vi "Instructor.vi"() -> ()   [LabVIEW 2017]
uses:
  <vilib>/Analysis/baseanly.llb/Mean (DBL).vi
  <vilib>/Utility/file.llb/Read Delimited Spreadsheet (DBL).vi
  <vilib>/Analysis/NI_AALBase.lvlib
panel:
  in  "error in (no error)":errorcluster
  in  "Desired Power":bool
  in  "Desired Power_S":sgl format="%#.1f"
  in  "TCHXActive":bool
  in  "PowerActive":bool
  in  "CTAHActive":bool
  in  "PumpActive":bool
  in  "ACTIVATE - TCHX_S":bool
  in  "ACTIVATE - PUMP_S":bool
  in  "ACTIVATE - CTAH_S":bool
  in  "Power Output On_S":bool
  in  "TCHXFreq_S":sgl format="%#.1f"
  in  "TCHXFreq":bool
  in  "Power_S":sgl format="%#.1f"
  in  "Power":bool
  in  "CTAHFreq_S":sgl format="%#.1f"
  in  "CTAHFreq":bool
  in  "PumpFreq_S":sgl format="%#.1f"
  in  "PumpFreq":bool
  out "W":sgl format="%.1f"
  out "S":sgl format="%.1f"
  out "E":sgl format="%.1f"
  out "N":sgl format="%.1f"
  out "SW":sgl format="%.1f"
  out "SE":sgl format="%.1f"
  out "N":sgl format="%.1f"
  out "Server Connection":bool
  in  "B66":bool
  in  "W67":bool
  in  "B60":bool
  in  "W61":bool
  in  "B65":bool
  in  "W64":bool
  in  "B21":bool
  in  "W20":bool
  in  "B23":bool
  in  "W22":bool
  in  "B63":bool
  in  "W62":bool
  in  "A01":bool
  in  "A02":bool
  in  "W24":bool
  in  "B25":bool
  in  "W26":bool
  in  "B27":bool
  in  "B12":bool
  in  "W13":bool
  in  "C11":bool
  in  "C10":bool
  in  "S13":bool
  in  "S11":bool
  in  "S10":bool
  in  "W35":bool
  in  "B34":bool
  in  "B43":bool
  in  "W42":bool
  in  "W40":bool
  in  "B41":bool
  in  "W33":bool
  in  "B32":bool
  in  "W31":bool
  in  "B30":bool
  in  "W10":bool
  in  "B11":bool
  in  "B29":bool
  in  "W28":bool
  in  "Spoof Enabled":bool
  in  "Stop Instructor":bool
  in  "BT-63_S":sgl format="%.1g"
  in  "WT-35_S":sgl format="%.1g"
  in  "BT-34_S":sgl format="%.1g"
  in  "ST-13_S":sgl format="%.1g"
  in  "ST-11_S":sgl format="%.1g"
  in  "ST-10_S":sgl format="%.1g"
  in  "BT-29_S":sgl format="%.1g"
  in  "BT-60_S":sgl format="%.1g"
  in  "AT-02_S":sgl format="%.1g"
  in  "AT-01_S":sgl format="%.1g"
  in  "BT-30_S":sgl format="%.1g"
  in  "BT-66_S":sgl format="%.1g"
  in  "BT-65_S":sgl format="%.1g"
  in  "BT-21_S":sgl format="%.1g"
  in  "BT-23_S":sgl format="%.1g"
  in  "BT-25_S":sgl format="%.1g"
  in  "BT-27_S":sgl format="%.1g"
  in  "BT-32_S":sgl format="%.1g"
  in  "BT-43_S":sgl format="%.1g"
  in  "BT-41_S":sgl format="%.1g"
  in  "WT-67_S":sgl format="%.1g"
  in  "WT-61_S":sgl format="%.1g"
  in  "WT-64_S":sgl format="%.1g"
  in  "WT-62_S":sgl format="%.1g"
  in  "WT-20_S":sgl format="%.1g"
  in  "WT-22_S":sgl format="%.1g"
  in  "WT-33_S":sgl format="%.1g"
  in  "WT-24_S":sgl format="%.1g"
  in  "WT-26_S":sgl format="%.1g"
  in  "WT-28_S":sgl format="%.1g"
  in  "WT-42_S":sgl format="%.1g"
  in  "WT-40_S":sgl format="%.1g"
  in  "WT-31_S":sgl format="%.1g"
  in  "BT-12_S":sgl format="%.1g"
  in  "BT-11_S":sgl format="%.1g"
  in  "WT-10_S":sgl format="%.1g"
  in  "CX-11_S":sgl format="%.1g"
  in  "CX-10_S":sgl format="%.1g"
  out "DRACS Flow\n\n\nFM-60 [kg/s]":sgl format="%.3f"
  out "Primary Flow\n\n\nFM-40 [kg/s]":sgl format="%.3f"
  out "Bypass Flow\n\n\nFM-30 [kg/s]":sgl format="%.3f"
  out "DHX Primary Flow\n\n\nFM-20 [kg/s]":sgl format="%.3f"
  out "AT-02":sgl format="%.1g"
  out "AT-01":sgl format="%.1g"
  out "ST-13":sgl format="%.1f"
  out "ST-11":sgl format="%.1f"
  out "ST-10":sgl format="%.1f"
  out "WT-67":sgl format="%.1f"
  out "BT-66":sgl format="%.1f"
  out "BT-65":sgl format="%.1f"
  out "WT-64":sgl format="%.1f"
  out "BT-63":sgl format="%.1f"
  out "WT-62":sgl format="%.1f"
  out "WT-61":sgl format="%.1f"
  out "BT-60":sgl format="%.1f"
  out "BT-43":sgl format="%.1g"
  out "WT-42":sgl format="%.1g"
  out "BT-41":sgl format="%.1g"
  out "WT-40":sgl format="%.1g"
  out "WT-35":sgl format="%.1g"
  out "BT-34":sgl format="%.1g"
  out "WT-33":sgl format="%.1g"
  out "BT-32":sgl format="%.1g"
  out "WT-31":sgl format="%.1g"
  out "BT-30":sgl format="%.1g"
  out "BT-29":sgl format="%.1f"
  out "WT-28":sgl format="%.1f"
  out "BT-27":sgl format="%.1f"
  out "WT-26":sgl format="%.1f"
  out "BT-25":sgl format="%.1f"
  out "WT-24":sgl format="%.1f"
  out "BT-23":sgl format="%.1f"
  out "WT-22":sgl format="%.1f"
  out "BT-21":sgl format="%.1f"
  out "WT-20":sgl format="%.1f"
  out "CX-11":sgl format="%.1g"
  out "CX-10":sgl format="%.1g"
  out "WT-13":sgl format="%.1g"
  out "BT-12":sgl format="%.1g"
  out "BT-11":sgl format="%.1g"
  out "WT-10":sgl format="%.1g"
  out "Power [W]":sgl(slide) caption="Power Output [W]" scale=0.0..10000.0
  out "Frequency [Hz]":sgl(knob) scale=0.0..45.0
  out "Frequency [Hz] 3":sgl(slide) scale=0.0..60.0
  out "Frequency [Hz]":sgl(slide) scale=0.0..60.0
  in  "WT-13_S":sgl format="%.1g"
  out "Power Output":sgl(graph)
  out "System Safe":bool
  out "System Time [s]":sgl format="%#.1f"
  out "System Loop Time (ms)":u32
  in  "Load Power Profile":bool
  in  "Dyn. Power Profile File":path
  out "CTAH Temperatures":cluster{"CTAH Outlet":dbl, "CTAH Inlet":dbl}(graph)
  out "CTAH Outlet":dbl format="%0.2f"
  out "CTAH Inlet":dbl format="%0.2f"
  out "Core Temperatures":cluster{"Heater Inlet":dbl, "Heater Outlet":dbl}(graph)
  out "Heater Outlet":dbl format="%0.2f"
  out "Heater Inlet":dbl format="%0.2f"
  out "Profile Step":i32
  out "Power Input Signal [W]":dbl
  out "Output Current 2 [A]":dbl
  out "Output Voltage 2 [V]":dbl
  out "Output Current 1 [A]":dbl
  out "Output Voltage 1 [V]":dbl
  out "Loop Period [ms]":i64
  # "System Analytics"
  # "DRACS"
  # "PRIMARY"
  # "HOT DRACS"
  # "DHX TOP"
  # "TCHX"
  # "HOT LEG"
  # "DHX"
  # "COLD DRACS"
  # "ST-14"
  # "BYPASS"
  # "CTAH"
  # "ST-12"
  # "DHX BOTTOM"
  # "HEATER"
  # "COLD LEG"
  # "PUMP"
  # "Action Log"
  # "Action Log Box"
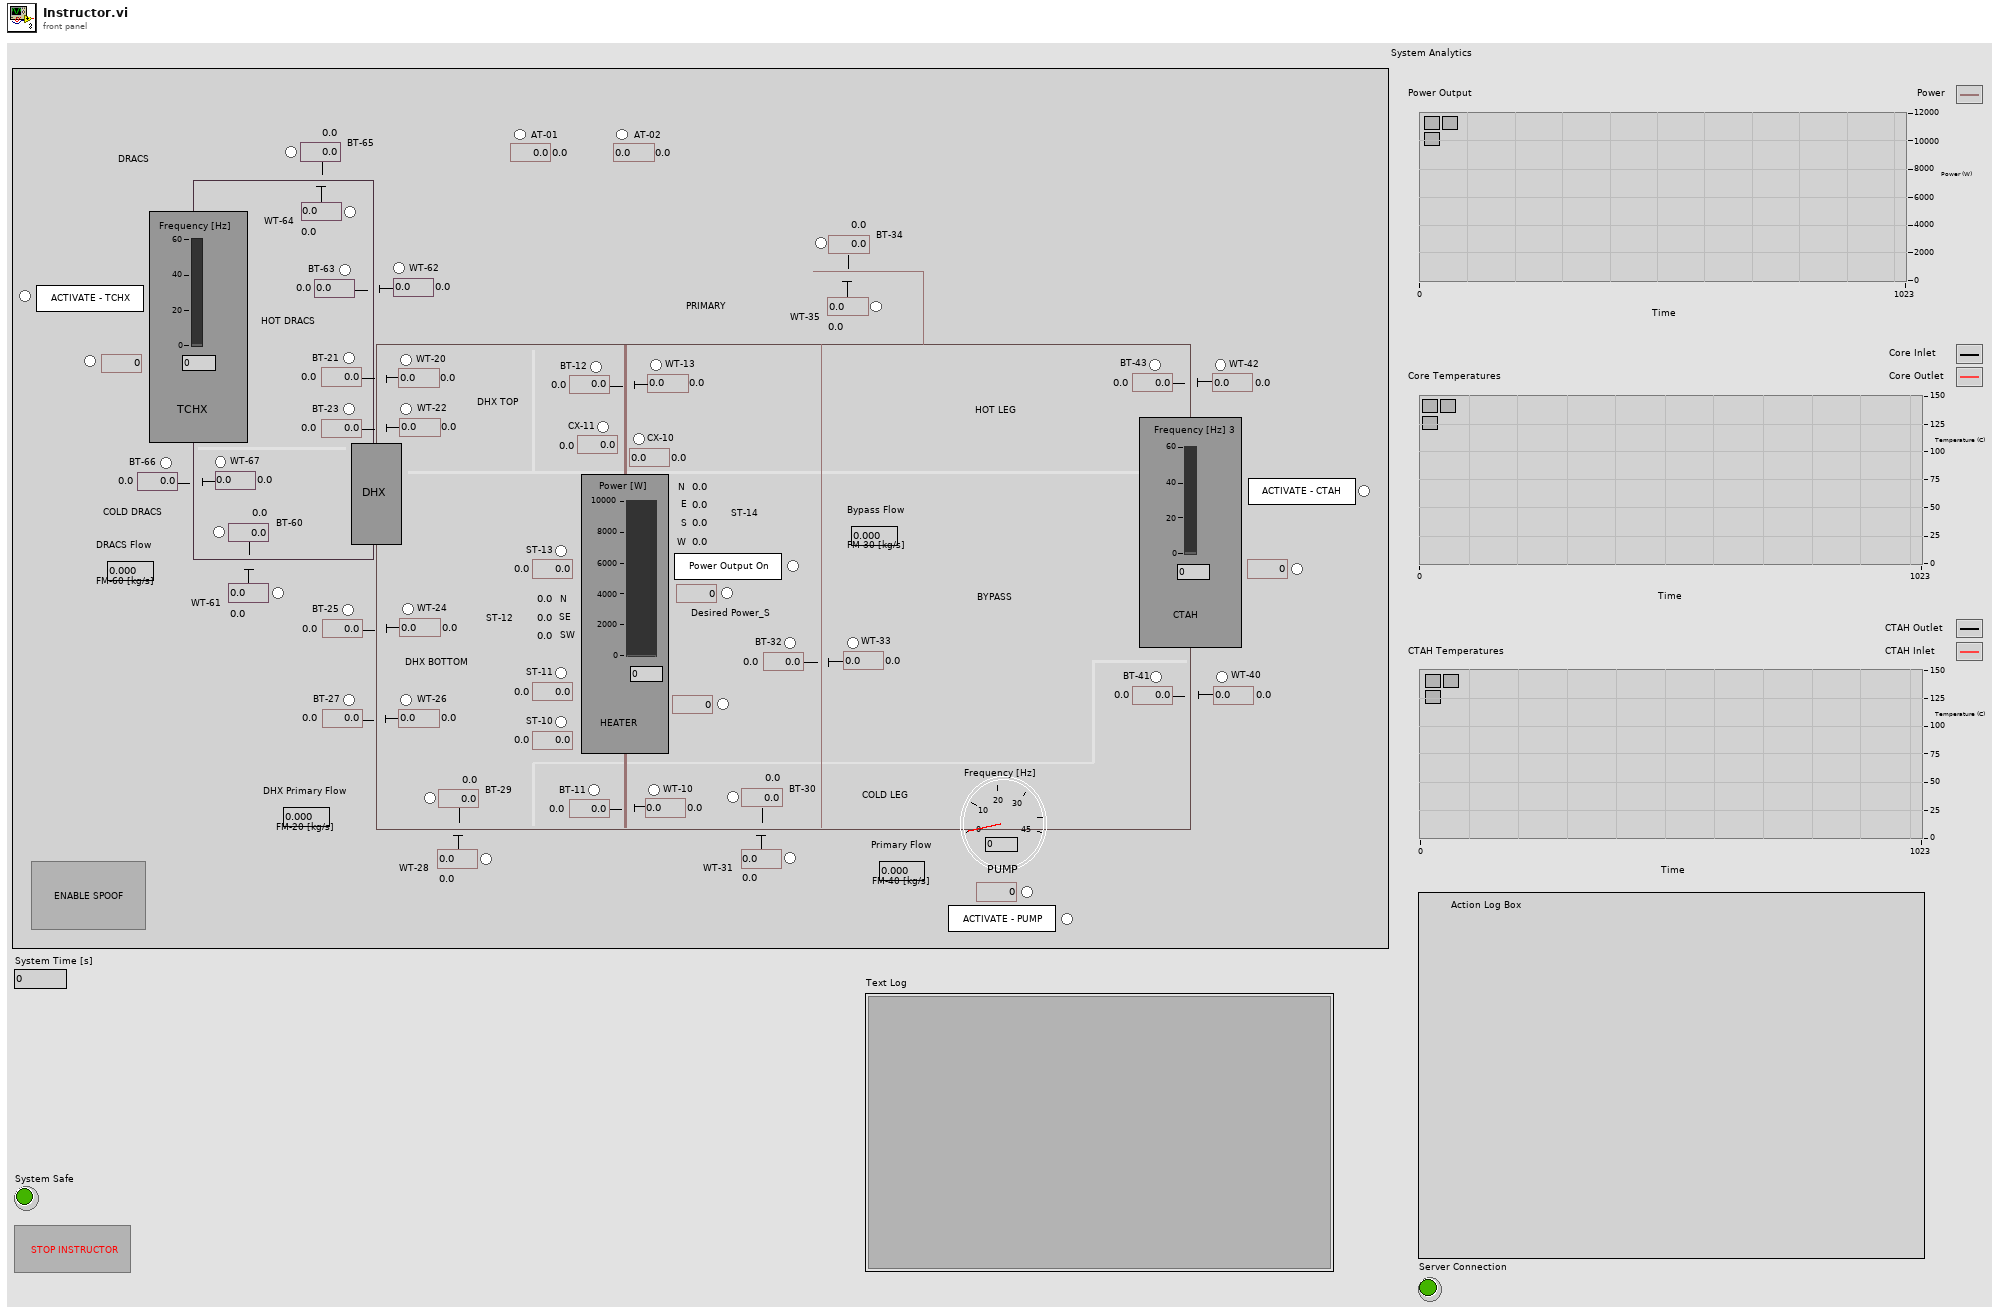
[diagram p1: front panel]
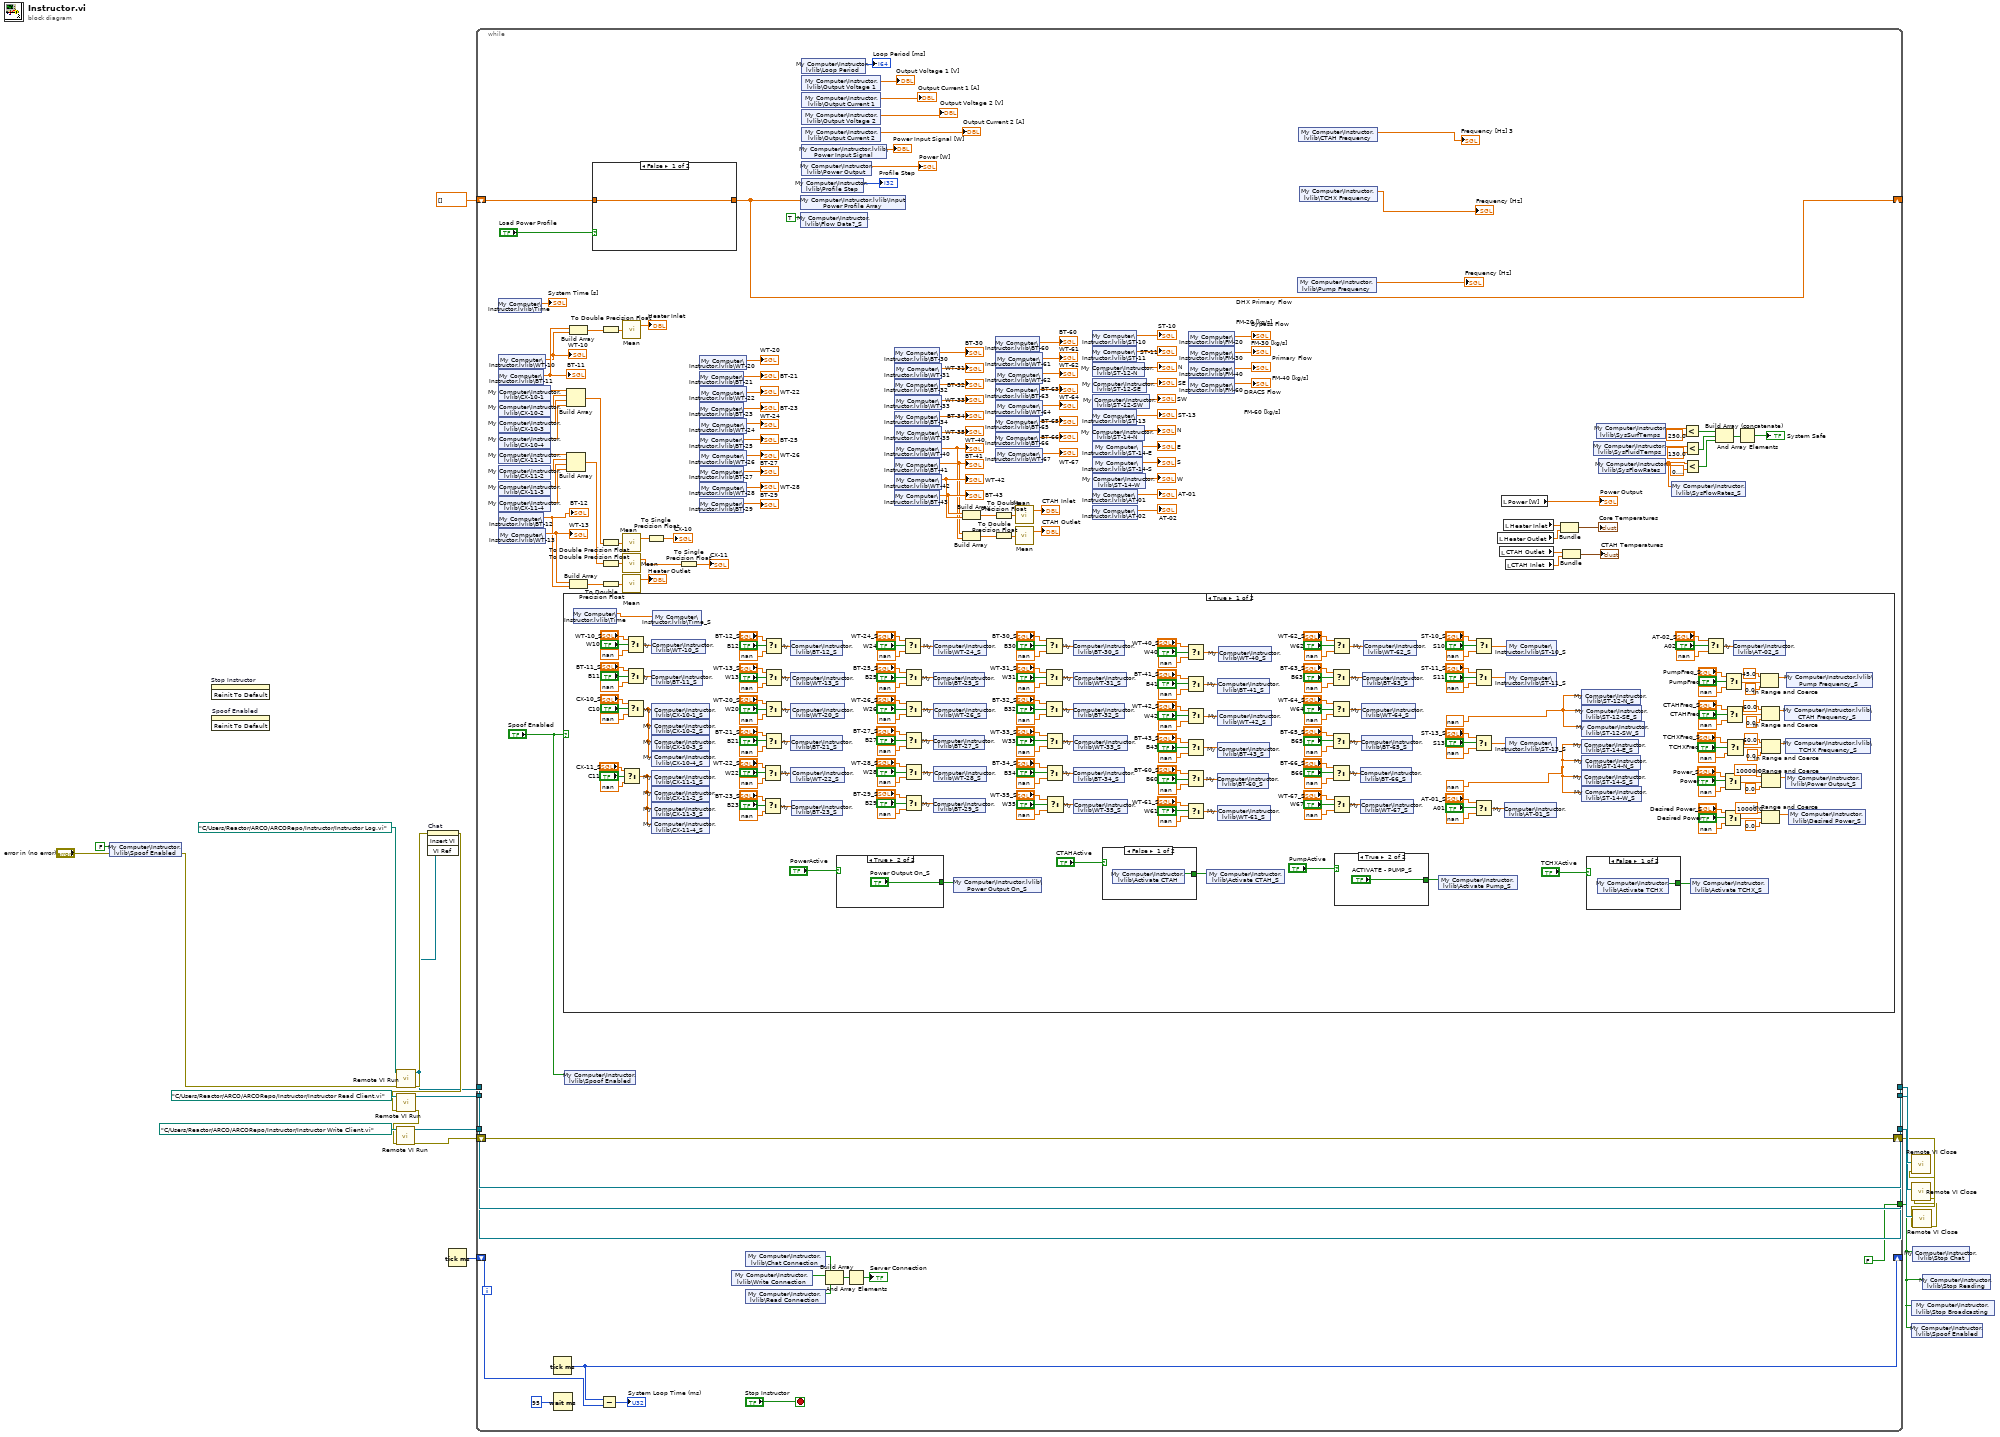
[diagram p0: block diagram]
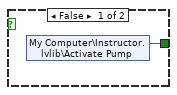
[diagram p2: hidden frame]
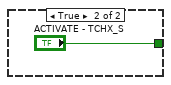
[diagram p3: hidden frame]
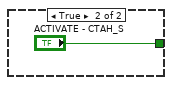
[diagram p4: hidden frame]
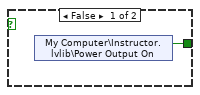
[diagram p5: hidden frame]
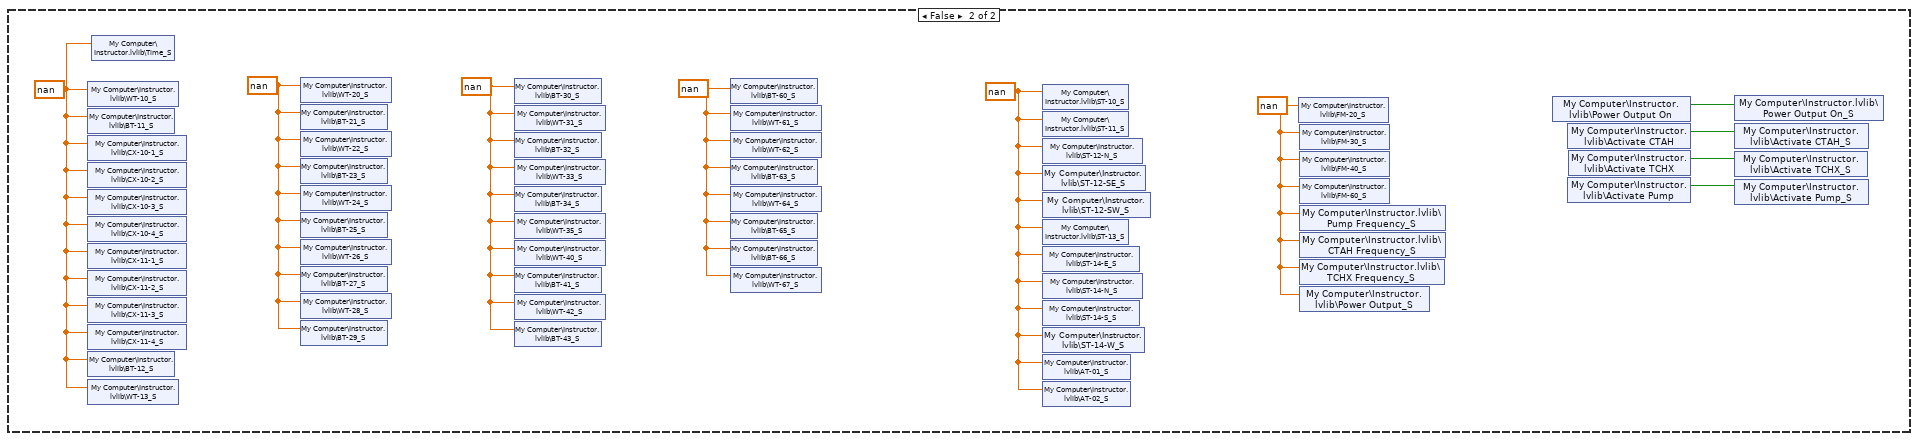
[diagram p6: hidden frame]
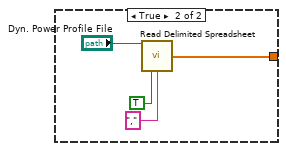
[diagram p7: hidden frame]
diagram:
  n1 = shared-variable "My Computer\\Instructor.lvlib\\Spoof Enabled"(FALSE ("Spoof Enabled"), error in="error in (no error)") -> (error out=w10:errorcluster)
  n2 = invoke on="Stop Instructor" class="Bool (strict)" method="Reinit To Default"() -> ()  [unwired: 3 in, 3 out]
  n3 = invoke on="Spoof Enabled" class="Bool (strict)" method="Reinit To Default"() -> ()  [unwired: 3 in, 3 out]
  n4 = call "Remote VI Run.vi"("error in (no error)"=w10, "VI Path"=path "C:/Users/Reactor/ARCO/ARCORepo/Instructor/Instructor Log.vi" ("vi path")) -> ("error out"=w9:errorcluster, "VI Reference"=w7:refnum<vi>)  [unwired: 8 in]
  n5 = invoke on="Chat" class="SubPnl" method="Insert VI"(error in=w9, "VI Ref"=w7) -> (error out=w8:errorcluster)  [unwired: 2 in, 3 out]
  n6 = call "Remote VI Run.vi"("error in (no error)"=w8, "VI Path"=path "C:/Users/Reactor/ARCO/ARCORepo/Instructor/Instructor Read Client.vi") -> ("error out"=w6:errorcluster, "VI Reference"=w18:refnum<vi>)  [unwired: 8 in]
  n7 = call "Remote VI Run.vi"("error in (no error)"=w6, "VI Path"=path "C:/Users/Reactor/ARCO/ARCORepo/Instructor/Instructor Write Client.vi") -> ("error out"=w5:errorcluster, "VI Reference"=w14:refnum<vi>)  [unwired: 8 in]
  n8 = Tick Count (ms)() -> (millisecond timer value=w21:u32)
  n9 = while {
    shift-right: [w73] -> _
    shift-left: dbl[] [] ("Input Power Profile Array") -> [w74]
    shift-right: [w71] -> _
    shift-left: w21 -> [w72]
    tunnel: w7 -> [w45]
    tunnel: w18 -> [w44]
    tunnel: [w45] -> w17
    tunnel: [w44] -> w16
    tunnel: w14 -> [w43]
    tunnel: [w43] -> w13
    tunnel: [FALSE] -> w12
    shift-right: [w24] -> w4
    shift-left: w5 -> [w24]
    stop <- "Stop Instructor" stop-if-true
    n10 = shared-variable "My Computer\\Instructor.lvlib\\Time"() -> (→"System Time [s]":sgl)  [unwired: 1 in, 1 out]
    n11 = shared-variable "My Computer\\Instructor.lvlib\\WT-10"() -> (w52:sgl)  [unwired: 1 in, 1 out]
    "WT-10" <- w52
    n12 = shared-variable "My Computer\\Instructor.lvlib\\BT-11"() -> (w56:sgl)  [unwired: 1 in, 1 out]
    "BT-11" <- w56
    n13 = shared-variable "My Computer\\Instructor.lvlib\\CX-10-1"() -> (w139:sgl)  [unwired: 1 in, 1 out]
    n14 = shared-variable "My Computer\\Instructor.lvlib\\CX-10-2"() -> (w138:sgl)  [unwired: 1 in, 1 out]
    n15 = shared-variable "My Computer\\Instructor.lvlib\\CX-10-3"() -> (w137:sgl)  [unwired: 1 in, 1 out]
    n16 = shared-variable "My Computer\\Instructor.lvlib\\CX-10-4"() -> (w136:sgl)  [unwired: 1 in, 1 out]
    n17 = shared-variable "My Computer\\Instructor.lvlib\\CX-11-1"() -> (w132:sgl)  [unwired: 1 in, 1 out]
    n18 = shared-variable "My Computer\\Instructor.lvlib\\CX-11-2"() -> (w131:sgl)  [unwired: 1 in, 1 out]
    n19 = shared-variable "My Computer\\Instructor.lvlib\\CX-11-3"() -> (w130:sgl)  [unwired: 1 in, 1 out]
    n20 = shared-variable "My Computer\\Instructor.lvlib\\CX-11-4"() -> (w129:sgl)  [unwired: 1 in, 1 out]
    n21 = shared-variable "My Computer\\Instructor.lvlib\\BT-12"() -> (w55:sgl)  [unwired: 1 in, 1 out]
    "BT-12" <- w55
    n22 = shared-variable "My Computer\\Instructor.lvlib\\WT-13"() -> (w96:sgl)  [unwired: 1 in, 1 out]
    "WT-13" <- w96
    n23 = Tick Count (ms)() -> (millisecond timer value=w71:u32)
    n24 = Wait (ms)(milliseconds to wait=u32 95) -> ()  [unwired: 1 out]
    n25 = case shown="True" "Spoof Enabled" {
      frame True {
        w192 = sgl nan
        w193 = sgl nan
        n26 = shared-variable "My Computer\\Instructor.lvlib\\Time"() -> (w194:sgl)  [unwired: 1 in, 1 out]
        n27 = Select(t="CX-11_S", s="C11", f=sgl nan) -> (s? t:f=w335:sgl)
        n28 = Select(t="WT-10_S", s="W10", f=sgl nan) -> (s? t:f=w347:sgl)
        n29 = Select(t="BT-11_S", s="B11", f=sgl nan) -> (s? t:f=w343:sgl)
        n30 = Select(t="CX-10_S", s="C10", f=sgl nan) -> (s? t:f=w339:sgl)
        n31 = shared-variable "My Computer\\Instructor.lvlib\\WT-10_S"(w347) -> ()  [unwired: 1 in, 1 out]
        n32 = shared-variable "My Computer\\Instructor.lvlib\\BT-11_S"(w343) -> ()  [unwired: 1 in, 1 out]
        n33 = shared-variable "My Computer\\Instructor.lvlib\\CX-10-1_S"(w339) -> ()  [unwired: 1 in, 1 out]
        n34 = shared-variable "My Computer\\Instructor.lvlib\\CX-10-2_S"(w339) -> ()  [unwired: 1 in, 1 out]
        n35 = shared-variable "My Computer\\Instructor.lvlib\\CX-10-3_S"(w339) -> ()  [unwired: 1 in, 1 out]
        n36 = shared-variable "My Computer\\Instructor.lvlib\\CX-10-4_S"(w339) -> ()  [unwired: 1 in, 1 out]
        n37 = shared-variable "My Computer\\Instructor.lvlib\\CX-11-1_S"(w335) -> ()  [unwired: 1 in, 1 out]
        n38 = shared-variable "My Computer\\Instructor.lvlib\\CX-11-2_S"(w335) -> ()  [unwired: 1 in, 1 out]
        n39 = shared-variable "My Computer\\Instructor.lvlib\\CX-11-3_S"(w335) -> ()  [unwired: 1 in, 1 out]
        n40 = shared-variable "My Computer\\Instructor.lvlib\\CX-11-4_S"(w335) -> ()  [unwired: 1 in, 1 out]
        n41 = shared-variable "My Computer\\Instructor.lvlib\\Time_S"(w194) -> ()  [unwired: 1 in, 1 out]
        n42 = Select(t="WT-22_S", s="W22", f=sgl nan) -> (s? t:f=w315:sgl)
        n43 = Select(t="BT-23_S", s="B23", f=sgl nan) -> (s? t:f=w311:sgl)
        n44 = Select(t="BT-12_S", s="B12", f=sgl nan) -> (s? t:f=w331:sgl)
        n45 = Select(t="WT-13_S", s="W13", f=sgl nan) -> (s? t:f=w327:sgl)
        n46 = Select(t="WT-20_S", s="W20", f=sgl nan) -> (s? t:f=w323:sgl)
        n47 = Select(t="BT-21_S", s="B21", f=sgl nan) -> (s? t:f=w319:sgl)
        n48 = shared-variable "My Computer\\Instructor.lvlib\\BT-12_S"(w331) -> ()  [unwired: 1 in, 1 out]
        n49 = shared-variable "My Computer\\Instructor.lvlib\\WT-13_S"(w327) -> ()  [unwired: 1 in, 1 out]
        n50 = shared-variable "My Computer\\Instructor.lvlib\\WT-20_S"(w323) -> ()  [unwired: 1 in, 1 out]
        n51 = shared-variable "My Computer\\Instructor.lvlib\\BT-21_S"(w319) -> ()  [unwired: 1 in, 1 out]
        n52 = shared-variable "My Computer\\Instructor.lvlib\\WT-22_S"(w315) -> ()  [unwired: 1 in, 1 out]
        n53 = shared-variable "My Computer\\Instructor.lvlib\\BT-23_S"(w311) -> ()  [unwired: 1 in, 1 out]
        n54 = case shown="True" "PowerActive" {
          tunnel: [w357 "Power Output On_S"] -> w155
          frame False {
            n55 = shared-variable "My Computer\\Instructor.lvlib\\Power Output On"() -> (w357:bool)  [unwired: 1 in, 1 out]
          }
          frame True {
          }
        }
        n56 = Select(t="WT-24_S", s="W24", f=sgl nan) -> (s? t:f=w307:sgl)
        n57 = Select(t="BT-25_S", s="B25", f=sgl nan) -> (s? t:f=w303:sgl)
        n58 = Select(t="WT-26_S", s="W26", f=sgl nan) -> (s? t:f=w299:sgl)
        n59 = Select(t="BT-27_S", s="B27", f=sgl nan) -> (s? t:f=w295:sgl)
        n60 = Select(t="WT-28_S", s="W28", f=sgl nan) -> (s? t:f=w291:sgl)
        n61 = Select(t="BT-29_S", s="B29", f=sgl nan) -> (s? t:f=w287:sgl)
        n62 = shared-variable "My Computer\\Instructor.lvlib\\WT-24_S"(w307) -> ()  [unwired: 1 in, 1 out]
        n63 = shared-variable "My Computer\\Instructor.lvlib\\BT-25_S"(w303) -> ()  [unwired: 1 in, 1 out]
        n64 = shared-variable "My Computer\\Instructor.lvlib\\WT-26_S"(w299) -> ()  [unwired: 1 in, 1 out]
        n65 = shared-variable "My Computer\\Instructor.lvlib\\BT-27_S"(w295) -> ()  [unwired: 1 in, 1 out]
        n66 = shared-variable "My Computer\\Instructor.lvlib\\WT-28_S"(w291) -> ()  [unwired: 1 in, 1 out]
        n67 = shared-variable "My Computer\\Instructor.lvlib\\BT-29_S"(w287) -> ()  [unwired: 1 in, 1 out]
        n68 = shared-variable "My Computer\\Instructor.lvlib\\Power Output On_S"(w155) -> ()  [unwired: 1 in, 1 out]
        n69 = Select(t="BT-30_S", s="B30", f=sgl nan) -> (s? t:f=w283:sgl)
        n70 = Select(t="WT-31_S", s="W31", f=sgl nan) -> (s? t:f=w279:sgl)
        n71 = Select(t="BT-32_S", s="B32", f=sgl nan) -> (s? t:f=w275:sgl)
        n72 = Select(t="WT-33_S", s="W33", f=sgl nan) -> (s? t:f=w271:sgl)
        n73 = Select(t="BT-34_S", s="B34", f=sgl nan) -> (s? t:f=w267:sgl)
        n74 = Select(t="WT-35_S", s="W35", f=sgl nan) -> (s? t:f=w263:sgl)
        n75 = shared-variable "My Computer\\Instructor.lvlib\\WT-31_S"(w279) -> ()  [unwired: 1 in, 1 out]
        n76 = shared-variable "My Computer\\Instructor.lvlib\\BT-32_S"(w275) -> ()  [unwired: 1 in, 1 out]
        n77 = shared-variable "My Computer\\Instructor.lvlib\\BT-30_S"(w283) -> ()  [unwired: 1 in, 1 out]
        n78 = shared-variable "My Computer\\Instructor.lvlib\\WT-33_S"(w271) -> ()  [unwired: 1 in, 1 out]
        n79 = shared-variable "My Computer\\Instructor.lvlib\\BT-34_S"(w267) -> ()  [unwired: 1 in, 1 out]
        n80 = shared-variable "My Computer\\Instructor.lvlib\\WT-35_S"(w263) -> ()  [unwired: 1 in, 1 out]
        n81 = case shown="False" "CTAHActive" {
          tunnel: [w355 "ACTIVATE - CTAH_S"] -> w153
          frame False {
            n82 = shared-variable "My Computer\\Instructor.lvlib\\Activate CTAH"() -> (w355:bool)  [unwired: 1 in, 1 out]
          }
          frame True {
          }
        }
        n83 = Select(t="WT-40_S", s="W40", f=sgl nan) -> (s? t:f=w259:sgl)
        n84 = Select(t="BT-41_S", s="B41", f=sgl nan) -> (s? t:f=w255:sgl)
        n85 = Select(t="WT-42_S", s="W42", f=sgl nan) -> (s? t:f=w251:sgl)
        n86 = Select(t="BT-43_S", s="B43", f=sgl nan) -> (s? t:f=w247:sgl)
        n87 = Select(t="BT-60_S", s="B60", f=sgl nan) -> (s? t:f=w243:sgl)
        n88 = Select(t="WT-61_S", s="W61", f=sgl nan) -> (s? t:f=w239:sgl)
        n89 = shared-variable "My Computer\\Instructor.lvlib\\Activate CTAH_S"(w153) -> ()  [unwired: 1 in, 1 out]
        n90 = shared-variable "My Computer\\Instructor.lvlib\\BT-60_S"(w243) -> ()  [unwired: 1 in, 1 out]
        n91 = shared-variable "My Computer\\Instructor.lvlib\\WT-61_S"(w239) -> ()  [unwired: 1 in, 1 out]
        n92 = shared-variable "My Computer\\Instructor.lvlib\\BT-41_S"(w255) -> ()  [unwired: 1 in, 1 out]
        n93 = shared-variable "My Computer\\Instructor.lvlib\\WT-42_S"(w251) -> ()  [unwired: 1 in, 1 out]
        n94 = shared-variable "My Computer\\Instructor.lvlib\\BT-43_S"(w247) -> ()  [unwired: 1 in, 1 out]
        n95 = shared-variable "My Computer\\Instructor.lvlib\\WT-40_S"(w259) -> ()  [unwired: 1 in, 1 out]
        n96 = Select(t="BT-63_S", s="B63", f=sgl nan) -> (s? t:f=w231:sgl)
        n97 = Select(t="WT-64_S", s="W64", f=sgl nan) -> (s? t:f=w227:sgl)
        n98 = Select(t="BT-65_S", s="B65", f=sgl nan) -> (s? t:f=w223:sgl)
        n99 = Select(t="BT-66_S", s="B66", f=sgl nan) -> (s? t:f=w219:sgl)
        n100 = Select(t="WT-62_S", s="W62", f=sgl nan) -> (s? t:f=w235:sgl)
        n101 = Select(t="WT-67_S", s="W67", f=sgl nan) -> (s? t:f=w215:sgl)
        n102 = case shown="True" "PumpActive" {
          tunnel: [w351 "ACTIVATE - PUMP_S"] -> w149
          frame False {
            n103 = shared-variable "My Computer\\Instructor.lvlib\\Activate Pump"() -> (w351:bool)  [unwired: 1 in, 1 out]
          }
          frame True {
          }
        }
        n104 = shared-variable "My Computer\\Instructor.lvlib\\WT-67_S"(w215) -> ()  [unwired: 1 in, 1 out]
        n105 = shared-variable "My Computer\\Instructor.lvlib\\BT-66_S"(w219) -> ()  [unwired: 1 in, 1 out]
        n106 = shared-variable "My Computer\\Instructor.lvlib\\BT-65_S"(w223) -> ()  [unwired: 1 in, 1 out]
        n107 = shared-variable "My Computer\\Instructor.lvlib\\WT-64_S"(w227) -> ()  [unwired: 1 in, 1 out]
        n108 = shared-variable "My Computer\\Instructor.lvlib\\BT-63_S"(w231) -> ()  [unwired: 1 in, 1 out]
        n109 = shared-variable "My Computer\\Instructor.lvlib\\WT-62_S"(w235) -> ()  [unwired: 1 in, 1 out]
        n110 = shared-variable "My Computer\\Instructor.lvlib\\Activate Pump_S"(w149) -> ()  [unwired: 1 in, 1 out]
        n111 = Select(t="ST-11_S", s="S11", f=sgl nan) -> (s? t:f=w207:sgl)
        n112 = Select(t="ST-13_S", s="S13", f=sgl nan) -> (s? t:f=w203:sgl)
        n113 = Select(t="AT-01_S", s="A01", f=sgl nan) -> (s? t:f=w199:sgl)
        n114 = Select(t="ST-10_S", s="S10", f=sgl nan) -> (s? t:f=w211:sgl)
        n115 = shared-variable "My Computer\\Instructor.lvlib\\AT-01_S"(w199) -> ()  [unwired: 1 in, 1 out]
        n116 = shared-variable "My Computer\\Instructor.lvlib\\ST-11_S"(w207) -> ()  [unwired: 1 in, 1 out]
        n117 = shared-variable "My Computer\\Instructor.lvlib\\ST-13_S"(w203) -> ()  [unwired: 1 in, 1 out]
        n118 = shared-variable "My Computer\\Instructor.lvlib\\ST-10_S"(w211) -> ()  [unwired: 1 in, 1 out]
        n119 = shared-variable "My Computer\\Instructor.lvlib\\ST-12-N_S"(w193) -> ()  [unwired: 1 in, 1 out]
        n120 = shared-variable "My Computer\\Instructor.lvlib\\ST-12-SE_S"(w193) -> ()  [unwired: 1 in, 1 out]
        n121 = shared-variable "My Computer\\Instructor.lvlib\\ST-12-SW_S"(w193) -> ()  [unwired: 1 in, 1 out]
        n122 = shared-variable "My Computer\\Instructor.lvlib\\ST-14-E_S"(w192) -> ()  [unwired: 1 in, 1 out]
        n123 = shared-variable "My Computer\\Instructor.lvlib\\ST-14-N_S"(w192) -> ()  [unwired: 1 in, 1 out]
        n124 = shared-variable "My Computer\\Instructor.lvlib\\ST-14-S_S"(w192) -> ()  [unwired: 1 in, 1 out]
        n125 = shared-variable "My Computer\\Instructor.lvlib\\ST-14-W_S"(w192) -> ()  [unwired: 1 in, 1 out]
        n126 = case shown="False" "TCHXActive" {
          tunnel: [w353 "ACTIVATE - TCHX_S"] -> w151
          frame False {
            n127 = shared-variable "My Computer\\Instructor.lvlib\\Activate TCHX"() -> (w353:bool)  [unwired: 1 in, 1 out]
          }
          frame True {
          }
        }
        n128 = shared-variable "My Computer\\Instructor.lvlib\\Activate TCHX_S"(w151) -> ()  [unwired: 1 in, 1 out]
        n129 = Select(t="AT-02_S", s="A02", f=sgl nan) -> (s? t:f=w195:sgl)
        n130 = Select(t="Power_S", s="Power", f=sgl nan) -> (s? t:f=w164:sgl)
        n131 = Select(t="Desired Power_S", s="Desired Power", f=sgl nan) -> (s? t:f=w161:sgl)
        n132 = Select(t="PumpFreq_S", s="PumpFreq", f=sgl nan) -> (s? t:f=w186:sgl)
        n133 = Select(t="CTAHFreq_S", s="CTAHFreq", f=sgl nan) -> (s? t:f=w182:sgl)
        n134 = Select(t="TCHXFreq_S", s="TCHXFreq", f=sgl nan) -> (s? t:f=w175:sgl)
        n135 = shared-variable "My Computer\\Instructor.lvlib\\AT-02_S"(w195) -> ()  [unwired: 1 in, 1 out]
        n136 = In Range and Coerce(upper limit=sgl 45.0, x=w186, lower limit=sgl 0.0) -> (coerced(x)=w185:sgl)  [unwired: 1 out]
        n137 = In Range and Coerce(upper limit=sgl 60.0, x=w182, lower limit=sgl 0.0) -> (coerced(x)=w178:sgl)  [unwired: 1 out]
        n138 = In Range and Coerce(upper limit=sgl 10000.0, x=w161, lower limit=sgl 0.0) -> (coerced(x)=w160:sgl)  [unwired: 1 out]
        n139 = In Range and Coerce(upper limit=sgl 60.0, x=w175, lower limit=sgl 0.0) -> (coerced(x)=w171:sgl)  [unwired: 1 out]
        n140 = In Range and Coerce(upper limit=sgl 10000.0, x=w164, lower limit=sgl 0.0) -> (coerced(x)=w159:sgl)  [unwired: 1 out]
        n141 = shared-variable "My Computer\\Instructor.lvlib\\CTAH Frequency_S"(w178) -> ()  [unwired: 1 in, 1 out]
        n142 = shared-variable "My Computer\\Instructor.lvlib\\TCHX Frequency_S"(w171) -> ()  [unwired: 1 in, 1 out]
        n143 = shared-variable "My Computer\\Instructor.lvlib\\Power Output_S"(w159) -> ()  [unwired: 1 in, 1 out]
        n144 = shared-variable "My Computer\\Instructor.lvlib\\Pump Frequency_S"(w185) -> ()  [unwired: 1 in, 1 out]
        n145 = shared-variable "My Computer\\Instructor.lvlib\\Desired Power_S"(w160) -> ()  [unwired: 1 in, 1 out]
      }
      frame False {
        w363 = sgl nan
        w365 = sgl nan
        w366 = sgl nan
        w367 = sgl nan
        w368 = sgl nan
        w364 = sgl nan
        n146 = shared-variable "My Computer\\Instructor.lvlib\\WT-10_S"(w364) -> ()  [unwired: 1 in, 1 out]
        n147 = shared-variable "My Computer\\Instructor.lvlib\\BT-11_S"(w364) -> ()  [unwired: 1 in, 1 out]
        n148 = shared-variable "My Computer\\Instructor.lvlib\\CX-10-1_S"(w364) -> ()  [unwired: 1 in, 1 out]
        n149 = shared-variable "My Computer\\Instructor.lvlib\\CX-10-2_S"(w364) -> ()  [unwired: 1 in, 1 out]
        n150 = shared-variable "My Computer\\Instructor.lvlib\\CX-10-3_S"(w364) -> ()  [unwired: 1 in, 1 out]
        n151 = shared-variable "My Computer\\Instructor.lvlib\\CX-10-4_S"(w364) -> ()  [unwired: 1 in, 1 out]
        n152 = shared-variable "My Computer\\Instructor.lvlib\\CX-11-1_S"(w364) -> ()  [unwired: 1 in, 1 out]
        n153 = shared-variable "My Computer\\Instructor.lvlib\\CX-11-2_S"(w364) -> ()  [unwired: 1 in, 1 out]
        n154 = shared-variable "My Computer\\Instructor.lvlib\\CX-11-3_S"(w364) -> ()  [unwired: 1 in, 1 out]
        n155 = shared-variable "My Computer\\Instructor.lvlib\\CX-11-4_S"(w364) -> ()  [unwired: 1 in, 1 out]
        n156 = shared-variable "My Computer\\Instructor.lvlib\\BT-12_S"(w364) -> ()  [unwired: 1 in, 1 out]
        n157 = shared-variable "My Computer\\Instructor.lvlib\\WT-13_S"(w364) -> ()  [unwired: 1 in, 1 out]
        n158 = shared-variable "My Computer\\Instructor.lvlib\\Time_S"(w364) -> ()  [unwired: 1 in, 1 out]
        n159 = shared-variable "My Computer\\Instructor.lvlib\\WT-20_S"(w368) -> ()  [unwired: 1 in, 1 out]
        n160 = shared-variable "My Computer\\Instructor.lvlib\\BT-21_S"(w368) -> ()  [unwired: 1 in, 1 out]
        n161 = shared-variable "My Computer\\Instructor.lvlib\\WT-22_S"(w368) -> ()  [unwired: 1 in, 1 out]
        n162 = shared-variable "My Computer\\Instructor.lvlib\\BT-23_S"(w368) -> ()  [unwired: 1 in, 1 out]
        n163 = shared-variable "My Computer\\Instructor.lvlib\\WT-24_S"(w368) -> ()  [unwired: 1 in, 1 out]
        n164 = shared-variable "My Computer\\Instructor.lvlib\\BT-25_S"(w368) -> ()  [unwired: 1 in, 1 out]
        n165 = shared-variable "My Computer\\Instructor.lvlib\\WT-26_S"(w368) -> ()  [unwired: 1 in, 1 out]
        n166 = shared-variable "My Computer\\Instructor.lvlib\\BT-27_S"(w368) -> ()  [unwired: 1 in, 1 out]
        n167 = shared-variable "My Computer\\Instructor.lvlib\\WT-28_S"(w368) -> ()  [unwired: 1 in, 1 out]
        n168 = shared-variable "My Computer\\Instructor.lvlib\\BT-29_S"(w368) -> ()  [unwired: 1 in, 1 out]
        n169 = shared-variable "My Computer\\Instructor.lvlib\\BT-30_S"(w367) -> ()  [unwired: 1 in, 1 out]
        n170 = shared-variable "My Computer\\Instructor.lvlib\\WT-31_S"(w367) -> ()  [unwired: 1 in, 1 out]
        n171 = shared-variable "My Computer\\Instructor.lvlib\\BT-32_S"(w367) -> ()  [unwired: 1 in, 1 out]
        n172 = shared-variable "My Computer\\Instructor.lvlib\\WT-33_S"(w367) -> ()  [unwired: 1 in, 1 out]
        n173 = shared-variable "My Computer\\Instructor.lvlib\\BT-34_S"(w367) -> ()  [unwired: 1 in, 1 out]
        n174 = shared-variable "My Computer\\Instructor.lvlib\\WT-35_S"(w367) -> ()  [unwired: 1 in, 1 out]
        n175 = shared-variable "My Computer\\Instructor.lvlib\\WT-40_S"(w367) -> ()  [unwired: 1 in, 1 out]
        n176 = shared-variable "My Computer\\Instructor.lvlib\\BT-41_S"(w367) -> ()  [unwired: 1 in, 1 out]
        n177 = shared-variable "My Computer\\Instructor.lvlib\\WT-42_S"(w367) -> ()  [unwired: 1 in, 1 out]
        n178 = shared-variable "My Computer\\Instructor.lvlib\\BT-43_S"(w367) -> ()  [unwired: 1 in, 1 out]
        n179 = shared-variable "My Computer\\Instructor.lvlib\\BT-60_S"(w366) -> ()  [unwired: 1 in, 1 out]
        n180 = shared-variable "My Computer\\Instructor.lvlib\\WT-61_S"(w366) -> ()  [unwired: 1 in, 1 out]
        n181 = shared-variable "My Computer\\Instructor.lvlib\\WT-62_S"(w366) -> ()  [unwired: 1 in, 1 out]
        n182 = shared-variable "My Computer\\Instructor.lvlib\\BT-63_S"(w366) -> ()  [unwired: 1 in, 1 out]
        n183 = shared-variable "My Computer\\Instructor.lvlib\\WT-64_S"(w366) -> ()  [unwired: 1 in, 1 out]
        n184 = shared-variable "My Computer\\Instructor.lvlib\\BT-65_S"(w366) -> ()  [unwired: 1 in, 1 out]
        n185 = shared-variable "My Computer\\Instructor.lvlib\\BT-66_S"(w366) -> ()  [unwired: 1 in, 1 out]
        n186 = shared-variable "My Computer\\Instructor.lvlib\\WT-67_S"(w366) -> ()  [unwired: 1 in, 1 out]
        n187 = shared-variable "My Computer\\Instructor.lvlib\\ST-10_S"(w365) -> ()  [unwired: 1 in, 1 out]
        n188 = shared-variable "My Computer\\Instructor.lvlib\\ST-11_S"(w365) -> ()  [unwired: 1 in, 1 out]
        n189 = shared-variable "My Computer\\Instructor.lvlib\\ST-12-N_S"(w365) -> ()  [unwired: 1 in, 1 out]
        n190 = shared-variable "My Computer\\Instructor.lvlib\\ST-12-SE_S"(w365) -> ()  [unwired: 1 in, 1 out]
        n191 = shared-variable "My Computer\\Instructor.lvlib\\ST-12-SW_S"(w365) -> ()  [unwired: 1 in, 1 out]
        n192 = shared-variable "My Computer\\Instructor.lvlib\\ST-13_S"(w365) -> ()  [unwired: 1 in, 1 out]
        n193 = shared-variable "My Computer\\Instructor.lvlib\\ST-14-E_S"(w365) -> ()  [unwired: 1 in, 1 out]
        n194 = shared-variable "My Computer\\Instructor.lvlib\\ST-14-N_S"(w365) -> ()  [unwired: 1 in, 1 out]
        n195 = shared-variable "My Computer\\Instructor.lvlib\\ST-14-S_S"(w365) -> ()  [unwired: 1 in, 1 out]
        n196 = shared-variable "My Computer\\Instructor.lvlib\\ST-14-W_S"(w365) -> ()  [unwired: 1 in, 1 out]
        n197 = shared-variable "My Computer\\Instructor.lvlib\\AT-01_S"(w365) -> ()  [unwired: 1 in, 1 out]
        n198 = shared-variable "My Computer\\Instructor.lvlib\\AT-02_S"(w365) -> ()  [unwired: 1 in, 1 out]
        n199 = shared-variable "My Computer\\Instructor.lvlib\\FM-20_S"(w363) -> ()  [unwired: 1 in, 1 out]
        n200 = shared-variable "My Computer\\Instructor.lvlib\\FM-30_S"(w363) -> ()  [unwired: 1 in, 1 out]
        n201 = shared-variable "My Computer\\Instructor.lvlib\\FM-40_S"(w363) -> ()  [unwired: 1 in, 1 out]
        n202 = shared-variable "My Computer\\Instructor.lvlib\\FM-60_S"(w363) -> ()  [unwired: 1 in, 1 out]
        n203 = shared-variable "My Computer\\Instructor.lvlib\\Pump Frequency_S"(w363) -> ()  [unwired: 1 in, 1 out]
        n204 = shared-variable "My Computer\\Instructor.lvlib\\CTAH Frequency_S"(w363) -> ()  [unwired: 1 in, 1 out]
        n205 = shared-variable "My Computer\\Instructor.lvlib\\TCHX Frequency_S"(w363) -> ()  [unwired: 1 in, 1 out]
        n206 = shared-variable "My Computer\\Instructor.lvlib\\Power Output_S"(w363) -> ()  [unwired: 1 in, 1 out]
        n207 = shared-variable "My Computer\\Instructor.lvlib\\Power Output On"() -> (w362:bool)  [unwired: 1 in, 1 out]
        n208 = shared-variable "My Computer\\Instructor.lvlib\\Activate CTAH"() -> (w361:bool)  [unwired: 1 in, 1 out]
        n209 = shared-variable "My Computer\\Instructor.lvlib\\Activate Pump"() -> (w359:bool)  [unwired: 1 in, 1 out]
        n210 = shared-variable "My Computer\\Instructor.lvlib\\Activate TCHX"() -> (w360:bool)  [unwired: 1 in, 1 out]
        n211 = shared-variable "My Computer\\Instructor.lvlib\\Power Output On_S"(w362) -> ()  [unwired: 1 in, 1 out]
        n212 = shared-variable "My Computer\\Instructor.lvlib\\Activate CTAH_S"(w361) -> ()  [unwired: 1 in, 1 out]
        n213 = shared-variable "My Computer\\Instructor.lvlib\\Activate TCHX_S"(w360) -> ()  [unwired: 1 in, 1 out]
        n214 = shared-variable "My Computer\\Instructor.lvlib\\Activate Pump_S"(w359) -> ()  [unwired: 1 in, 1 out]
      }
    }
    n215 = shared-variable "My Computer\\Instructor.lvlib\\Spoof Enabled"("Spoof Enabled") -> ()  [unwired: 1 in, 1 out]
    n216 = Build Array(w139, w138, w137, w136) -> (w135:sgl[])
    n217 = Build Array(w132, w131, w130, w129) -> (w128:sgl[])
    n218 = Build Array(w56, w52) -> (w94:sgl[])
    n219 = Build Array(w96, w55) -> (w97:sgl[])
    n220 = case shown="False" "Load Power Profile" {
      tunnel: [w369 w370] -> w73
      tunnel: w74 -> [w369 _]
      frame False {
      }
      frame True {
        n221 = call-poly <vilib>:"Read Delimited Spreadsheet.vi"("file path (dialog if empty)"="Dyn. Power Profile File", "transpose? (F)"=TRUE, "delimiter (\\t)"="," ("delimiter (\\t)")) -> ("first row"=w370:dbl[])  [unwired: 7 in, 5 out]
      }
    }
    n222 = Subtract(x=w71, y=w72) -> (x-y=→"System Loop Time (ms)":u32)
    n223 = To Double Precision Float(number=w94) -> (double precision float=w95:dbl[])
    n224 = To Double Precision Float(number=w135) -> (double precision float=w134:dbl[])
    n225 = To Double Precision Float(number=w128) -> (double precision float=w133:dbl[])
    n226 = To Double Precision Float(number=w97) -> (double precision float=w98:dbl[])
    n227 = call-poly <vilib>:"Mean.vi"("X"=w95) -> ("mean"=→"Heater Inlet":dbl)  [unwired: 1 out]
    n228 = call-poly <vilib>:"Mean.vi"("X"=w134) -> ("mean"=w58:dbl)  [unwired: 1 out]
    n229 = call-poly <vilib>:"Mean.vi"("X"=w133) -> ("mean"=w57:dbl)  [unwired: 1 out]
    n230 = call-poly <vilib>:"Mean.vi"("X"=w98) -> ("mean"=→"Heater Outlet":dbl)  [unwired: 1 out]
    n231 = To Single Precision Float(number=w58) -> (single precision float=→"CX-10":sgl)
    n232 = To Single Precision Float(number=w57) -> (single precision float=→"CX-11":sgl)
    n233 = shared-variable "My Computer\\Instructor.lvlib\\WT-20"() -> (→"WT-20":sgl)  [unwired: 1 in, 1 out]
    n234 = shared-variable "My Computer\\Instructor.lvlib\\BT-21"() -> (→"BT-21":sgl)  [unwired: 1 in, 1 out]
    n235 = shared-variable "My Computer\\Instructor.lvlib\\WT-22"() -> (→"WT-22":sgl)  [unwired: 1 in, 1 out]
    n236 = shared-variable "My Computer\\Instructor.lvlib\\BT-23"() -> (→"BT-23":sgl)  [unwired: 1 in, 1 out]
    n237 = shared-variable "My Computer\\Instructor.lvlib\\WT-24"() -> (→"WT-24":sgl)  [unwired: 1 in, 1 out]
    n238 = shared-variable "My Computer\\Instructor.lvlib\\BT-25"() -> (→"BT-25":sgl)  [unwired: 1 in, 1 out]
    n239 = shared-variable "My Computer\\Instructor.lvlib\\WT-26"() -> (→"WT-26":sgl)  [unwired: 1 in, 1 out]
    n240 = shared-variable "My Computer\\Instructor.lvlib\\BT-27"() -> (→"BT-27":sgl)  [unwired: 1 in, 1 out]
    n241 = shared-variable "My Computer\\Instructor.lvlib\\WT-28"() -> (→"WT-28":sgl)  [unwired: 1 in, 1 out]
    n242 = shared-variable "My Computer\\Instructor.lvlib\\BT-29"() -> (→"BT-29":sgl)  [unwired: 1 in, 1 out]
    n243 = shared-variable "My Computer\\Instructor.lvlib\\Write Connection"() -> (w40:bool)  [unwired: 1 in, 1 out]
    n244 = shared-variable "My Computer\\Instructor.lvlib\\Read Connection"() -> (w39:bool)  [unwired: 1 in, 1 out]
    n245 = shared-variable "My Computer\\Instructor.lvlib\\Chat Connection"() -> (w41:bool)  [unwired: 1 in, 1 out]
    n246 = shared-variable "My Computer\\Instructor.lvlib\\Input Power Profile Array"(w73) -> ()  [unwired: 1 in, 1 out]
    n247 = shared-variable "My Computer\\Instructor.lvlib\\Flow Data?_S"(TRUE ("Flow Data?")) -> ()  [unwired: 1 in, 1 out]
    n248 = shared-variable "My Computer\\Instructor.lvlib\\Loop Period"() -> (→"Loop Period [ms]":i64)  [unwired: 1 in, 1 out]
    n249 = shared-variable "My Computer\\Instructor.lvlib\\Output Voltage 1"() -> (→"Output Voltage 1 [V]":dbl)  [unwired: 1 in, 1 out]
    n250 = shared-variable "My Computer\\Instructor.lvlib\\Output Current 1"() -> (→"Output Current 1 [A]":dbl)  [unwired: 1 in, 1 out]
    n251 = shared-variable "My Computer\\Instructor.lvlib\\Output Voltage 2"() -> (→"Output Voltage 2 [V]":dbl)  [unwired: 1 in, 1 out]
    n252 = shared-variable "My Computer\\Instructor.lvlib\\Output Current 2"() -> (→"Output Current 2 [A]":dbl)  [unwired: 1 in, 1 out]
    n253 = shared-variable "My Computer\\Instructor.lvlib\\Power Input Signal"() -> (→"Power Input Signal [W]":sgl)  [unwired: 1 in, 1 out]
    n254 = shared-variable "My Computer\\Instructor.lvlib\\Power Output"() -> (→"Power [W]":sgl)  [unwired: 1 in, 1 out]
    n255 = shared-variable "My Computer\\Instructor.lvlib\\Profile Step"() -> (→"Profile Step":i32)  [unwired: 1 in, 1 out]
    n256 = Build Array(w41, w40, w39) -> (w38:bool[])
    n257 = And Array Elements(Boolean array=w38) -> (logical AND=→"Server Connection":bool)
    n258 = shared-variable "My Computer\\Instructor.lvlib\\BT-30"() -> (→"BT-30":sgl)  [unwired: 1 in, 1 out]
    n259 = shared-variable "My Computer\\Instructor.lvlib\\WT-31"() -> (→"WT-31":sgl)  [unwired: 1 in, 1 out]
    n260 = shared-variable "My Computer\\Instructor.lvlib\\BT-32"() -> (→"BT-32":sgl)  [unwired: 1 in, 1 out]
    n261 = shared-variable "My Computer\\Instructor.lvlib\\WT-33"() -> (→"WT-33":sgl)  [unwired: 1 in, 1 out]
    n262 = shared-variable "My Computer\\Instructor.lvlib\\BT-34"() -> (→"BT-34":sgl)  [unwired: 1 in, 1 out]
    n263 = shared-variable "My Computer\\Instructor.lvlib\\WT-35"() -> (→"WT-35":sgl)  [unwired: 1 in, 1 out]
    n264 = shared-variable "My Computer\\Instructor.lvlib\\WT-40"() -> (w80:sgl)  [unwired: 1 in, 1 out]
    "WT-40" <- w80
    n265 = shared-variable "My Computer\\Instructor.lvlib\\BT-41"() -> (w79:sgl)  [unwired: 1 in, 1 out]
    "BT-41" <- w79
    n266 = shared-variable "My Computer\\Instructor.lvlib\\WT-42"() -> (w82:sgl)  [unwired: 1 in, 1 out]
    "WT-42" <- w82
    n267 = shared-variable "My Computer\\Instructor.lvlib\\BT-43"() -> (w81:sgl)  [unwired: 1 in, 1 out]
    "BT-43" <- w81
    n268 = Build Array(w81, w82) -> (w87:sgl[])
    n269 = Build Array(w79, w80) -> (w84:sgl[])
    n270 = shared-variable "My Computer\\Instructor.lvlib\\BT-60"() -> (→"BT-60":sgl)  [unwired: 1 in, 1 out]
    n271 = shared-variable "My Computer\\Instructor.lvlib\\WT-61"() -> (→"WT-61":sgl)  [unwired: 1 in, 1 out]
    n272 = shared-variable "My Computer\\Instructor.lvlib\\WT-62"() -> (→"WT-62":sgl)  [unwired: 1 in, 1 out]
    n273 = shared-variable "My Computer\\Instructor.lvlib\\BT-63"() -> (→"BT-63":sgl)  [unwired: 1 in, 1 out]
    n274 = shared-variable "My Computer\\Instructor.lvlib\\WT-64"() -> (→"WT-64":sgl)  [unwired: 1 in, 1 out]
    n275 = shared-variable "My Computer\\Instructor.lvlib\\BT-65"() -> (→"BT-65":sgl)  [unwired: 1 in, 1 out]
    n276 = shared-variable "My Computer\\Instructor.lvlib\\BT-66"() -> (→"BT-66":sgl)  [unwired: 1 in, 1 out]
    n277 = shared-variable "My Computer\\Instructor.lvlib\\WT-67"() -> (→"WT-67":sgl)  [unwired: 1 in, 1 out]
    n278 = To Double Precision Float(number=w87) -> (double precision float=w88:dbl[])
    n279 = To Double Precision Float(number=w84) -> (double precision float=w85:dbl[])
    n280 = call-poly <vilib>:"Mean.vi"("X"=w88) -> ("mean"=→"CTAH Inlet":dbl)  [unwired: 1 out]
    n281 = call-poly <vilib>:"Mean.vi"("X"=w85) -> ("mean"=→"CTAH Outlet":dbl)  [unwired: 1 out]
    n282 = shared-variable "My Computer\\Instructor.lvlib\\ST-10"() -> (→"ST-10":sgl)  [unwired: 1 in, 1 out]
    n283 = shared-variable "My Computer\\Instructor.lvlib\\ST-11"() -> (→"ST-11":sgl)  [unwired: 1 in, 1 out]
    n284 = shared-variable "My Computer\\Instructor.lvlib\\ST-12-N"() -> (→"N":sgl)  [unwired: 1 in, 1 out]
    n285 = shared-variable "My Computer\\Instructor.lvlib\\ST-12-SE"() -> (→"SE":sgl)  [unwired: 1 in, 1 out]
    n286 = shared-variable "My Computer\\Instructor.lvlib\\ST-12-SW"() -> (→"SW":sgl)  [unwired: 1 in, 1 out]
    n287 = shared-variable "My Computer\\Instructor.lvlib\\ST-13"() -> (→"ST-13":sgl)  [unwired: 1 in, 1 out]
    n288 = shared-variable "My Computer\\Instructor.lvlib\\ST-14-N"() -> (→"N":sgl)  [unwired: 1 in, 1 out]
    n289 = shared-variable "My Computer\\Instructor.lvlib\\ST-14-E"() -> (→"E":sgl)  [unwired: 1 in, 1 out]
    n290 = shared-variable "My Computer\\Instructor.lvlib\\ST-14-S"() -> (→"S":sgl)  [unwired: 1 in, 1 out]
    n291 = shared-variable "My Computer\\Instructor.lvlib\\ST-14-W"() -> (→"W":sgl)  [unwired: 1 in, 1 out]
    n292 = shared-variable "My Computer\\Instructor.lvlib\\AT-01"() -> (→"AT-01":sgl)  [unwired: 1 in, 1 out]
    n293 = shared-variable "My Computer\\Instructor.lvlib\\AT-02"() -> (→"AT-02":sgl)  [unwired: 1 in, 1 out]
    n294 = shared-variable "My Computer\\Instructor.lvlib\\FM-20"() -> (→"DHX Primary Flow\n\n\nFM-20 [kg/s]":sgl)  [unwired: 1 in, 1 out]
    n295 = shared-variable "My Computer\\Instructor.lvlib\\FM-30"() -> (→"Bypass Flow\n\n\nFM-30 [kg/s]":sgl)  [unwired: 1 in, 1 out]
    n296 = shared-variable "My Computer\\Instructor.lvlib\\FM-40"() -> (→"Primary Flow\n\n\nFM-40 [kg/s]":sgl)  [unwired: 1 in, 1 out]
    n297 = shared-variable "My Computer\\Instructor.lvlib\\FM-60"() -> (→"DRACS Flow\n\n\nFM-60 [kg/s]":sgl)  [unwired: 1 in, 1 out]
    n298 = shared-variable "My Computer\\Instructor.lvlib\\Pump Frequency"() -> (→"Frequency [Hz]":sgl)  [unwired: 1 in, 1 out]
    n299 = shared-variable "My Computer\\Instructor.lvlib\\CTAH Frequency"() -> (→"Frequency [Hz] 3":sgl)  [unwired: 1 in, 1 out]
    n300 = shared-variable "My Computer\\Instructor.lvlib\\TCHX Frequency"() -> (→"Frequency [Hz]":sgl)  [unwired: 1 in, 1 out]
    n301 = local read "Heater Outlet"() -> (w89:dbl)
    n302 = local read "CTAH Outlet"() -> (w77:dbl)
    n303 = local read "Power [W]"() -> (→"Power Output":sgl)
    n304 = local read "Heater Inlet"() -> (w90:dbl)
    n305 = local read "CTAH Inlet"() -> (w76:dbl)
    n306 = Bundle("Heater Inlet"=w90, "Heater Outlet"=w89) -> (→"Core Temperatures":cluster{"Heater Inlet":dbl, "Heater Outlet":dbl})  [unwired: 1 in]
    n307 = Bundle("CTAH Outlet"=w77, "CTAH Inlet"=w76) -> (→"CTAH Temperatures":cluster{"CTAH Outlet":dbl, "CTAH Inlet":dbl})  [unwired: 1 in]
    n308 = shared-variable "My Computer\\Instructor.lvlib\\SysFluidTemps"() -> (w64:sgl[])  [unwired: 1 in, 1 out]
    n309 = shared-variable "My Computer\\Instructor.lvlib\\SysSurfTemps"() -> (w66:sgl[])  [unwired: 1 in, 1 out]
    n310 = shared-variable "My Computer\\Instructor.lvlib\\SysFlowRates"() -> (w51:sgl[])  [unwired: 1 in, 1 out]
    n311 = shared-variable "My Computer\\Instructor.lvlib\\SysFlowRates_S"(w51) -> ()  [unwired: 1 in, 1 out]
    n312 = Less?(x=w66, y=sgl 250.0) -> (x < y?=w68:bool[])
    n313 = Less?(x=w64, y=sgl 130.0) -> (x < y?=w62:bool[])
    n314 = Less?(x=w51, y=sgl 0.2) -> (x < y?=w61:bool[])
    n315 = Build Array (concatenate)(w68, w62, w61) -> (w69:bool[])
    n316 = And Array Elements(Boolean array=w69) -> (logical AND=→"System Safe":bool)
  }
  n317 = shared-variable "My Computer\\Instructor.lvlib\\Stop Broadcasting"(w12) -> ()  [unwired: 1 in, 1 out]
  n318 = shared-variable "My Computer\\Instructor.lvlib\\Spoof Enabled"(w12) -> ()  [unwired: 1 in, 1 out]
  n319 = shared-variable "My Computer\\Instructor.lvlib\\Stop Chat"(w12) -> ()  [unwired: 1 in, 1 out]
  n320 = call "Remote VI Close.vi"("error in (no error)"=w4, "reference"=w13) -> ("error out"=w3:errorcluster)  [unwired: 8 in, 1 out]
  n321 = call "Remote VI Close.vi"("error in (no error)"=w3, "reference"=w16) -> ("error out"=w2:errorcluster)  [unwired: 8 in, 1 out]
  n322 = call "Remote VI Close.vi"("error in (no error)"=w2, "reference"=w17) -> ()  [unwired: 8 in, 2 out]
  n323 = shared-variable "My Computer\\Instructor.lvlib\\Stop Reading"(w12) -> ()  [unwired: 1 in, 1 out]
